vi "sv_Concatenate Label and Unit.vi"(4 "unit string":string, 5 "label":string) -> (1 "scale label with units":string)   [LabVIEW 2017]
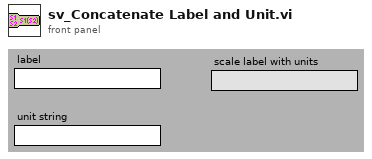
[diagram p1: front panel]
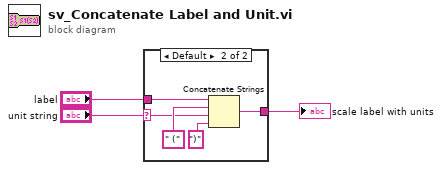
[diagram p0: block diagram]
diagram:
  n1 = case shown="Default" "unit string" {
    selector: "unit string" -> [_ w5]
    tunnel: [w4 w9] -> w3
    tunnel: "label" -> [w4 w8]
    frame "" {
    }
    frame Default {
      n2 = Concatenate Strings(w8, " (" ("string"), w5, ")" ("string")) -> (w9:string)
    }
  }
  "scale label with units" <- w3
